vi "Color_Sensor.vi"(11 "MotorControlDevRef":T1={"DeviceStatus"={"status"=FALSE, "code"=0, "source"=""}, "Type"=enum."PWM", "PWM"={"PWM Channel"=enum."Invalid", "DeadBand"={"Name"="", "maxPositivePwm"=0, "minPositivePwm"=0, "centerPwm"=0, "maxNegativePwm"=0, "minNegativePwm"=0, "angularRange"=0}}, "CAN"={"Device Number"=0, "SetOutput VI Ref"=variant(refnum<vi> refnum), "GetOutput VI Ref"=variant(refnum<vi> refnum), "Enable VI Ref"=variant(refnum<vi> refnum), "Disable VI Ref"=variant(refnum<vi> refnum), "Data"=variant}, "Invert"=FALSE, "DIO PWM"={"PWM \"Enable\" Channel"=enum."Invalid", "DIOChannel"=enum."Invalid", "PWM Rate"=0.0}}) -> ()   [LabVIEW 2019]
uses:
  <vilib>/Rock Robotics/WPI/ThirdParty/REV Robotics/SPARK MAX/Typedef/Spark MAX Control Type.ctl
  <vilib>/Rock Robotics/SystemInterfaces/DIO/FPGA_DIOPWMChannel.ctl
  <vilib>/Rock Robotics/WPI/PWM/WPI_PWMDeadband.ctl
  <vilib>/Rock Robotics/WPI/MotorControl/WPI_MotorControlType.ctl
  <vilib>/Rock Robotics/SystemInterfaces/DIO/FPGA_DIOChannel.ctl
  <vilib>/Rock Robotics/WPI/MotorControl/WPI_MotorControlDeviceRef.ctl
panel:
  out "Color Match? 2":bool
  out "Matched Color Name 2":string
  out "Match Confidence 2":dbl
  out "Measured Color 2":cluster{"R":dbl, "G":dbl, "B":dbl}
  out "error out 2":errorcluster
  out "Proximity 2":u16(graph)
  out "Color 2":u32(colorbox)
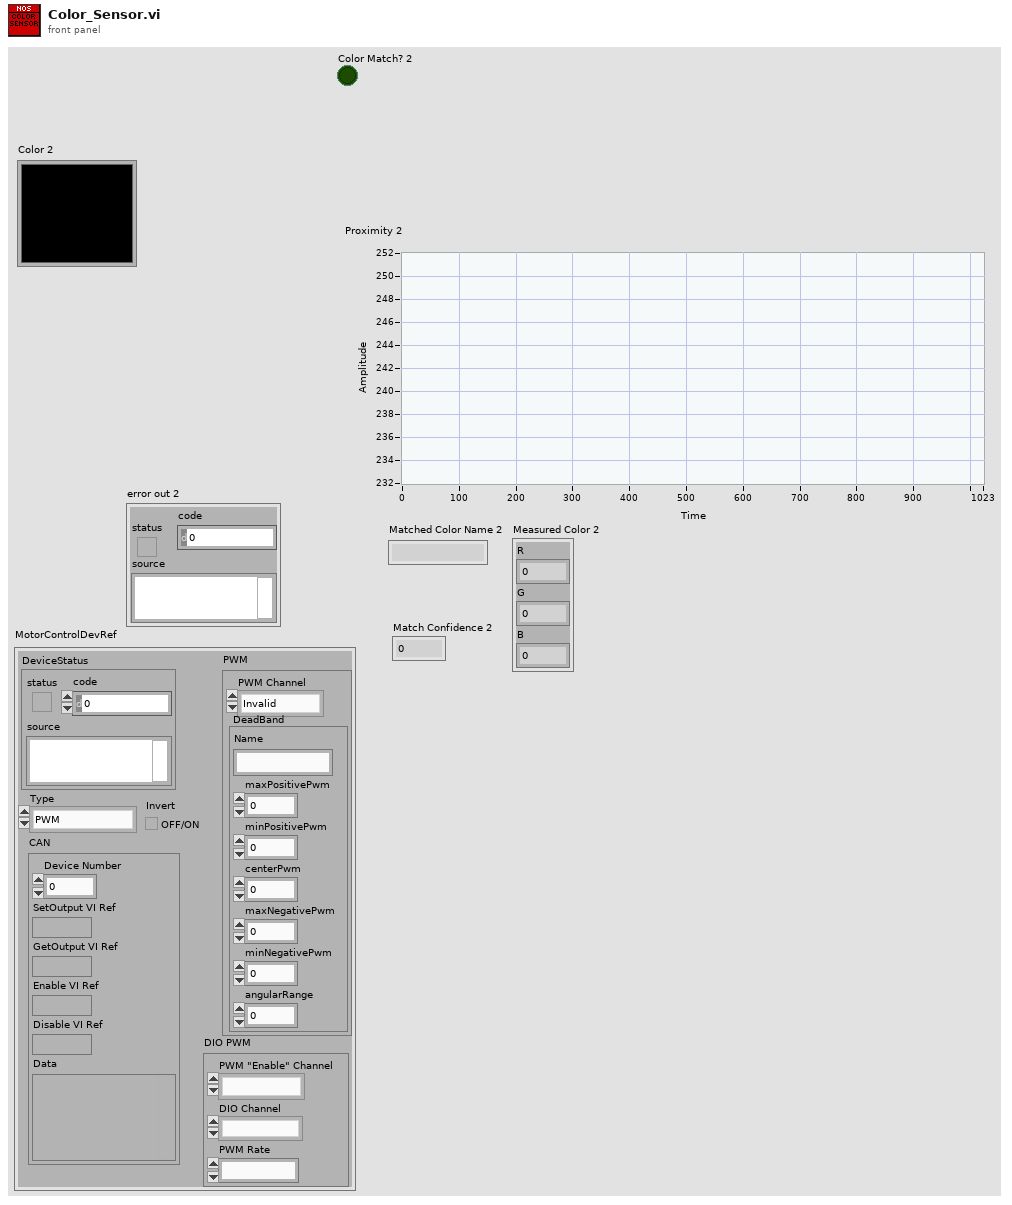
[diagram p1: front panel]
types:
  T1 = typedef "WPI_MotorControlDeviceRef.ctl" = cluster{"DeviceStatus":errorcluster, "Type":T2, "PWM":cluster{"PWM Channel":T3, "DeadBand":T4}, "CAN":cluster{"Device Number":u8, "SetOutput VI Ref":variant, "GetOutput VI Ref":variant, "Enable VI Ref":variant, "Disable VI Ref":variant, "Data":variant}, "Invert":bool, "DIO PWM":cluster{"PWM \"Enable\" Channel":T3, "DIOChannel":T5, "PWM Rate":dbl}}
  T2 = typedef "WPI_MotorControlType.ctl" = enum16{"PWM", "CAN", "DIO PWM"}
  T3 = typedef "FPGA_DIOPWMChannel.ctl" = enum8{"PWM 0", "PWM 1", "PWM 2", "PWM 3", "PWM 4", "PWM 5", "PWM 6", "PWM 7", "PWM 8", "PWM 9", "PWM MXP 0", "PWM MXP 1", "PWM MXP 2", "PWM MXP 3", "PWM MXP 4", "PWM MXP 5", "PWM MXP 6", "PWM MXP 7", "PWM MXP 8", "PWM MXP 9", "Invalid"}
  T4 = typedef "WPI_PWMDeadband.ctl" = cluster{"Name":string, "maxPositivePwm":i32, "minPositivePwm":i32, "centerPwm":i32, "maxNegativePwm":i32, "minNegativePwm":i32, "angularRange":u16}
  T5 = typedef "FPGA_DIOChannel.ctl" = enum8{"DIO 0", "DIO 1", "DIO 2", "DIO 3", "DIO 4", "DIO 5", "DIO 6", "DIO 7", "DIO 8", "DIO 9", "DIO MXP 0", "DIO MXP 1", "DIO MXP 2", "DIO MXP 3", "DIO MXP 4", "DIO MXP 5", "DIO MXP 6", "DIO MXP 7", "DIO MXP 8", "DIO MXP 9", "DIO MXP 10", "DIO MXP 11", "DIO MXP 12", "DIO MXP 13", "DIO MXP 14", "DIO MXP 15", "SPI Port CS1", "SPI Port CS2", "SPI Port CS3", "SPI Port MISO", "SPI Port MOSI", "Invalid"}
  T6 = typedef "Spark MAX Control Type.ctl" = enum16{"Percent VBus", "Voltage", "Velocity", "Position", "Smart Motion", "Current", "Smart Velocity"}
  T7 = typedef "Color Sensor V3 DevRef.ctl" = cluster{"I2CDevRef":T8}
  T8 = typedef "WPI_I2CDevRef.ctl" = cluster{"DevStatus":errorcluster, "Device Address":u8, "Handle":i32, "I2C Bus":T9}
  T9 = typedef "i2c_bus.ctl" = enum16{"I2C On-Board", "I2C MXP", "Invalid"}
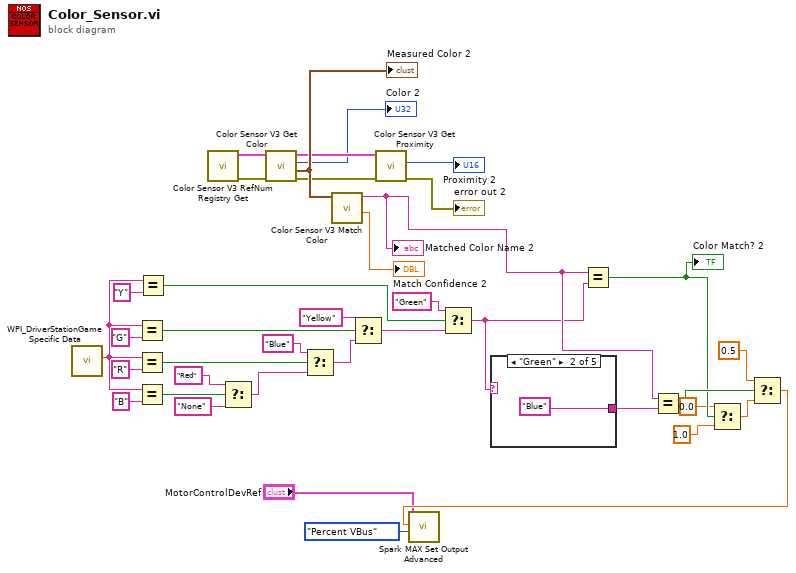
[diagram p0: block diagram]
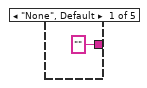
[diagram p2: hidden frame]
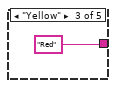
[diagram p3: hidden frame]
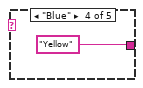
[diagram p4: hidden frame]
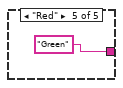
[diagram p5: hidden frame]
diagram:
  n1 = call <vilib>:"WPI_DriverStationGame Specific Data.vi"() -> ("Game Specific Data"=w23:string)  [unwired: 11 in]
  n2 = Equal?(x=w23, y="G") -> (x = y?=w28:bool)
  n3 = Equal?(x=w23, y="R") -> (x = y?=w25:bool)
  n4 = Equal?(x=w23, y="B") -> (x = y?=w24:bool)
  n5 = Equal?(x=w23, y="Y") -> (x = y?=w30:bool)
  n6 = call <vilib>:"Color Sensor V3 RefNum Registry Get.vi"() -> ("error out"=w31:errorcluster, "ColorSensorDevRef"=w32:T7)  [unwired: 10 in]
  n7 = Select(t="Red" ("Color"), s=w24, f="None") -> (s? t:f=w26:string)
  n8 = call <vilib>:"Color Sensor V3 Get Color.vi"("error in (no error)"=w31, "ColorSensorDevRef"=w32) -> ("error out"=w17:errorcluster, "Normalized Color"=w21:cluster{"R":dbl, "G":dbl, "B":dbl}, "Color"=→"Color 2":u32, "ColorSensorDevRef out"=w18:T7)  [unwired: 6 in]
  "Measured Color 2" <- w21
  n9 = Select(t="Blue", s=w25, f=w26) -> (s? t:f=w27:string)
  n10 = call <vilib>:"Color Sensor V3 Match Color.vi"("Measured Color"=w21) -> ("Confidence"=→"Match Confidence 2":dbl, "Matched Color Name"=w36:string)  [unwired: 8 in, 1 out]
  "Matched Color Name 2" <- w36
  n11 = Select(t="Yellow", s=w28, f=w27) -> (s? t:f=w29:string)
  n12 = call <vilib>:"Color Sensor V3 Get Proximity.vi"("error in (no error)"=w17, "ColorSensorDevRef"=w18) -> ("error out"=→"error out 2":errorcluster, "Proximity"=→"Proximity 2":u16)  [unwired: 7 in, 1 out]
  n13 = Select(t="Green", s=w30, f=w29) -> (s? t:f=w34:string)
  n14 = case shown="\"Green\"" w34 {
    tunnel: ["" ("t") "Blue" ("t") "Red" ("t") "Yellow" ("t") "Green" ("t")] -> w35
    frame "None", Default {
    }
    frame "Green" {
    }
    frame "Yellow" {
    }
    frame "Blue" {
    }
    frame "Red" {
    }
  }
  n15 = Equal?(x=w36, y=w34) -> (x = y?=w33:bool)
  "Color Match? 2" <- w33
  n16 = Equal?(x=w36, y=w35) -> (x = y?=w38:bool)
  n17 = Select(t=0.0, s=w33, f=1.0 ("Output")) -> (s? t:f=w37:dbl)
  n18 = Select(t=0.5, s=w38, f=w37) -> (s? t:f=w2:dbl)
  n19 = call <vilib>:"Spark MAX Set Output Advanced.vi"("Control Mode"=Spark_MAX_Control_Type."Percent VBus", "Setpoint"=w2, "MotorControlDevRef"="MotorControlDevRef") -> ()  [unwired: 7 in, 2 out]
